vi "isScriptAvailable.vi"(8 "error in (no error)":errorcluster, 11 "ExperimentRunner in":refnum<class "ExperimentRunner.lvclass">) -> (0 "error out":errorcluster, 1 "available":bool, 2 "selectedScript":i32, 3 "ExperimentRunner out":refnum<class "ExperimentRunner.lvclass">)   [LabVIEW 2011, in "Views.lvlib" / "ExperimentControl.lvlib" / "ExperimentRunner.lvclass"]
uses:
  ExperimentRunner.lvclass
  ExperimentRunner.lvclass/ExperimentRunner.ctl
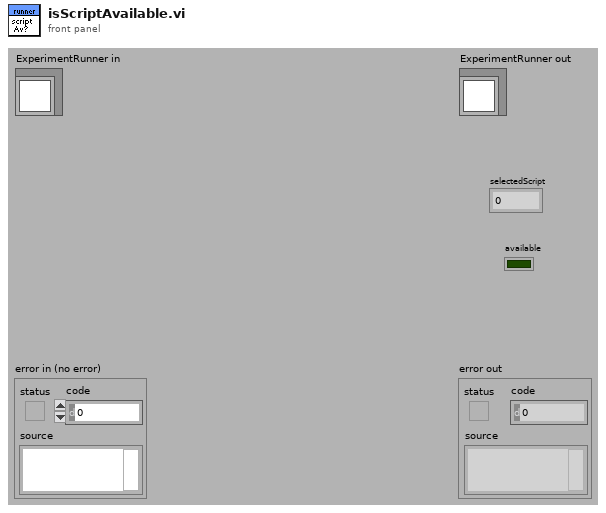
[diagram p1: front panel]
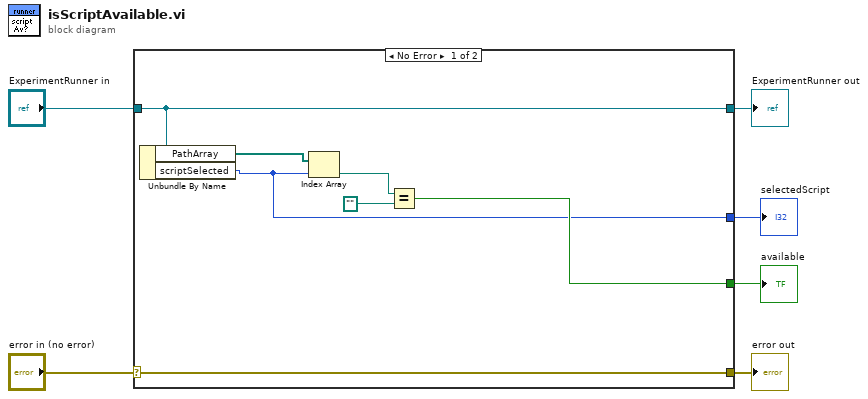
[diagram p0: block diagram]
diagram:
  n1 = case shown="No Error" "error in (no error)" {
    selector: "error in (no error)" -> [w13 w15]
    tunnel: [w13 w15] -> w5
    tunnel: [w12 w14] -> w3
    tunnel: "ExperimentRunner in" -> [w12 w14]
    tunnel: [w8 _] -> w2
    tunnel: [w7 _] -> w1
    frame No Error {
      n2 = Unbundle By Name(w12) -> ("PathArray"=w11:path[], "scriptSelected"=w7:i32)
      n3 = Index Array(array=w11, index=w7) -> (element=w9:path)
      n4 = Equal?(x=w9, y=path "") -> (x = y?=w8:bool)
    }
    frame Error {
    }
  }
  "error out" <- w5
  "ExperimentRunner out" <- w3
  "selectedScript" <- w1
  "available" <- w2
